vi "Read G08 Clock Params.vi"(8 "error in (no error)":errorcluster, 11 "BME_DG_G08 in":refnum<class "BME_DG_G08.lvclass">) -> (0 "error out":errorcluster, 1 "Trigger Multiplier":u32, 2 "Trigger Divider":u32, 3 "BME_DG_G08 out":refnum<class "BME_DG_G08.lvclass">)   [LabVIEW 2009, in "BME_DG_G08.lvclass"]
uses:
  BME_DG_G08.lvclass
  BME_DG_G08.lvclass/BME_DG_G08.ctl
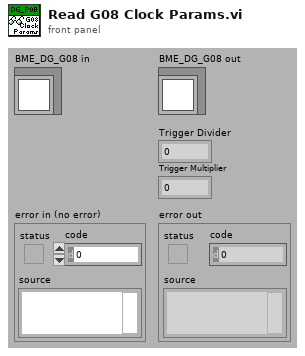
[diagram p1: front panel]
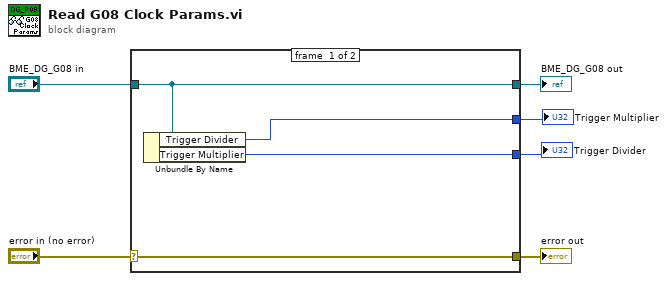
[diagram p0: block diagram]
diagram:
  n1 = case shown="No Error" "error in (no error)" {
    selector: "error in (no error)" -> [w10 w11]
    tunnel: [w10 w11] -> w5
    tunnel: [w9 w12] -> w3
    tunnel: "BME_DG_G08 in" -> [w9 w12]
    tunnel: [w8 _] -> w2
    tunnel: [w7 _] -> w1
    frame #0 {
      n2 = Unbundle By Name(w9) -> ("Trigger Divider"=w8:u32, "Trigger Multiplier"=w7:u32)
    }
    frame #1 {
    }
  }
  "error out" <- w5
  "BME_DG_G08 out" <- w3
  "Trigger Divider" <- w1
  "Trigger Multiplier" <- w2
